vi "CreateAllMessageQueues.vi"(8 "entrée d'erreur":errorcluster caption="entrée d'erreur (pas d'erreur)") -> (0 "error out":errorcluster, 3 "All Message Queue Cluster":T1)   [LabVIEW 2013, in "MessageQueues.lvlib"]
doc: "Ce VI crée et nomme les piles qui seront utilisées par le programme principale. Chaque pile correspond à un appareil ou un service (sous programme).\n\nentrée :\n-error : erreur d'entrée\n\nsortie :\n- All Message Queue cluster : cluster contenant toutes les piles utilisé par le programme principale.\n- error : erreur de sortie.\n\nCe VI contruit un cluster qui englobe toutes les entité \"queues\" qui seront utilisées par le VI principale\nIl est possible d'en rajouter en copiant le ligne \"obtain Queue.vi\" et \"AddMessage.vi\"\n\nLa dénomination des queues ce fait en modifiant le cluster \"All Message Queue cluster\" \ndepuis l'objet commande stric \"All message Queue cluster.ctl\""
uses:
  MessageQueues.lvlib
  AllMessageQueue Cluster.ctl
  Message Cluster.ctl
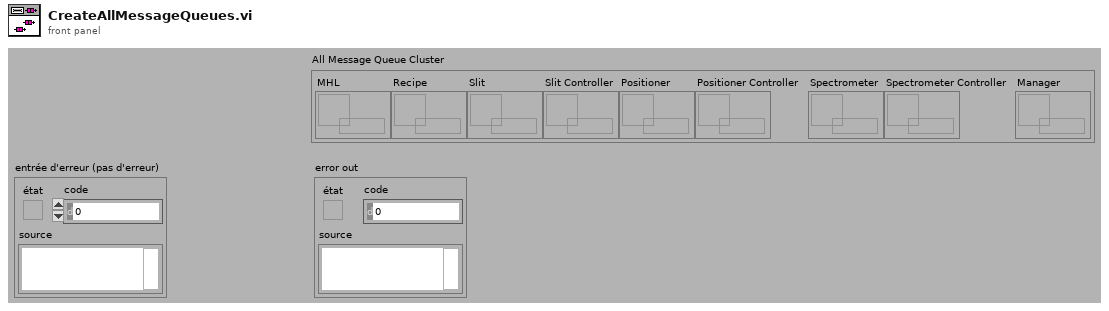
[diagram p1: front panel]
types:
  T1 = typedef "MessageQueues.lvlib/AllMessageQueue Cluster.ctl" = cluster{"MHL":refnum<queue>, "Recipe":refnum<queue>, "Slit":refnum<queue>, "Slit Controller":refnum<queue>, "Positioner":refnum<queue>, "Positioner Controller":refnum<queue>, "Spectrometer":refnum<queue>, "Spectrometer Controller":refnum<queue>, "Manager":refnum<queue>}
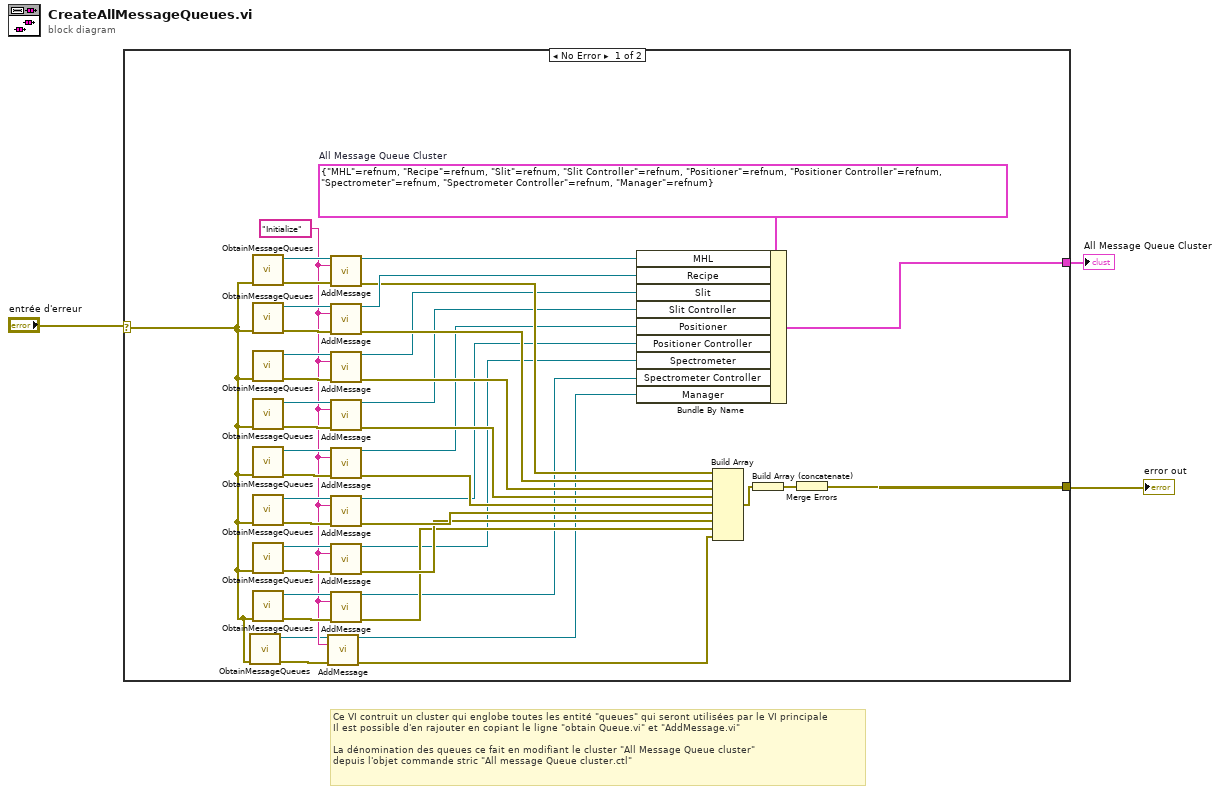
[diagram p0: block diagram]
diagram:
  # "Ce VI contruit un cluster qui englobe toutes les entité \"queues\" qui seront utilisées par le VI principale\nIl est possible d'en rajouter en copiant le ligne \"obtain Queue.vi\" et \"AddMessage.vi\"\n\nLa dénomination des queues ce fait en modifiant le cluster \"All Message Queue cluster\" \ndepuis l'objet commande stric \"All message Queue cluster.ctl\""
  n1 = case shown="No Error" "entrée d'erreur" {
    selector: "entrée d'erreur" -> [w7 w47]
    tunnel: [w37 w47] -> w2
    tunnel: [w36 _] -> w1
    frame No Error {
      w35 = T1 {"MHL"=refnum, "Recipe"=refnum, "Slit"=refnum, "Slit Controller"=refnum, "Positioner"=refnum, "Positioner Controller"=refnum, "Spectrometer"=refnum, "Spectrometer Controller"=refnum, "Manager"=refnum}  # All Message Queue Cluster
      w6 = "Initialize"
      n2 = call "ObtainMessageQueues.vi"("entrée d'erreur (pas d'erreur)"=w7) -> ("sortie d'erreur"=w9:errorcluster, "Message queue"=w4:refnum<queue>)  [unwired: 9 in]
      n3 = call "ObtainMessageQueues.vi"("entrée d'erreur (pas d'erreur)"=w7) -> ("sortie d'erreur"=w45:errorcluster, "Message queue"=w44:refnum<queue>)  [unwired: 9 in]
      n4 = call "ObtainMessageQueues.vi"("entrée d'erreur (pas d'erreur)"=w7) -> ("sortie d'erreur"=w46:errorcluster, "Message queue"=w43:refnum<queue>)  [unwired: 9 in]
      n5 = call "ObtainMessageQueues.vi"("entrée d'erreur (pas d'erreur)"=w7) -> ("sortie d'erreur"=w34:errorcluster, "Message queue"=w32:refnum<queue>)  [unwired: 9 in]
      n6 = call "ObtainMessageQueues.vi"("entrée d'erreur (pas d'erreur)"=w7) -> ("sortie d'erreur"=w33:errorcluster, "Message queue"=w31:refnum<queue>)  [unwired: 9 in]
      n7 = call "ObtainMessageQueues.vi"("entrée d'erreur (pas d'erreur)"=w7) -> ("sortie d'erreur"=w26:errorcluster, "Message queue"=w27:refnum<queue>)  [unwired: 9 in]
      n8 = call "ObtainMessageQueues.vi"("entrée d'erreur (pas d'erreur)"=w7) -> ("sortie d'erreur"=w25:errorcluster, "Message queue"=w24:refnum<queue>)  [unwired: 9 in]
      n9 = call "ObtainMessageQueues.vi"("entrée d'erreur (pas d'erreur)"=w7) -> ("sortie d'erreur"=w20:errorcluster, "Message queue"=w21:refnum<queue>)  [unwired: 9 in]
      n10 = call "ObtainMessageQueues.vi"("entrée d'erreur (pas d'erreur)"=w7) -> ("sortie d'erreur"=w19:errorcluster, "Message queue"=w18:refnum<queue>)  [unwired: 9 in]
      n11 = call "AddMessage.vi"("Message queue"=w4, "Message"=w6, "entrée d'erreur (pas d'erreur)"=w9) -> ("Dup Message queue"=w5:refnum<queue>, "error out"=w8:errorcluster)  [unwired: 11 in]
      n12 = call "AddMessage.vi"("Message queue"=w44, "Message"=w6, "entrée d'erreur (pas d'erreur)"=w45) -> ("Dup Message queue"=w41:refnum<queue>, "error out"=w40:errorcluster)  [unwired: 11 in]
      n13 = call "AddMessage.vi"("Message queue"=w43, "Message"=w6, "entrée d'erreur (pas d'erreur)"=w46) -> ("Dup Message queue"=w42:refnum<queue>, "error out"=w39:errorcluster)  [unwired: 11 in]
      n14 = call "AddMessage.vi"("Message queue"=w32, "Message"=w6, "entrée d'erreur (pas d'erreur)"=w34) -> ("Dup Message queue"=w15:refnum<queue>, "error out"=w30:errorcluster)  [unwired: 11 in]
      n15 = call "AddMessage.vi"("Message queue"=w31, "Message"=w6, "entrée d'erreur (pas d'erreur)"=w33) -> ("Dup Message queue"=w14:refnum<queue>, "error out"=w29:errorcluster)  [unwired: 11 in]
      n16 = call "AddMessage.vi"("Message queue"=w27, "Message"=w6, "entrée d'erreur (pas d'erreur)"=w26) -> ("Dup Message queue"=w13:refnum<queue>, "error out"=w22:errorcluster)  [unwired: 11 in]
      n17 = call "AddMessage.vi"("Message queue"=w24, "Message"=w6, "entrée d'erreur (pas d'erreur)"=w25) -> ("Dup Message queue"=w12:refnum<queue>, "error out"=w23:errorcluster)  [unwired: 11 in]
      n18 = call "AddMessage.vi"("Message queue"=w21, "Message"=w6, "entrée d'erreur (pas d'erreur)"=w20) -> ("Dup Message queue"=w11:refnum<queue>, "error out"=w17:errorcluster)  [unwired: 11 in]
      n19 = call "AddMessage.vi"("Message queue"=w18, "Message"=w6, "entrée d'erreur (pas d'erreur)"=w19) -> ("Dup Message queue"=w10:refnum<queue>, "error out"=w16:errorcluster)  [unwired: 11 in]
      n20 = Bundle By Name(cluster=w35, "MHL"=w41, "Recipe"=w42, "Slit"=w15, "Slit Controller"=w14, "Positioner"=w13, "Positioner Controller"=w12, "Spectrometer"=w11, "Spectrometer Controller"=w10, "Manager"=w5) -> (w36:T1)
      n21 = Build Array(w40, w39, w30, w29, w22, w23, w17, w16, w8) -> (w38:errorcluster[])
      n22 = Build Array (concatenate)(w38) -> (w28:errorcluster[])
      n23 = Merge Errors(w28) -> (w37:errorcluster)
    }
    frame Error {
    }
  }
  "error out" <- w2
  "All Message Queue Cluster" <- w1
